vi "Read U8 Array.vi"(8 "error in":errorcluster, 9 "size":i32, 10 "register name":string, 11 "session in":u32) -> (0 "error out":errorcluster, 2 "Value out":u8[](array[numeric]), 3 "session out":u32)   [LabVIEW 2020, in "FPGA Register IO.lvlib"]
uses:
  FPGA Register IO.lvlib
  SubVIs/Check Register Data Store.vi
  Error Handling/Error 6001.vi
  Error Handling/Error 6000.vi
  Error Handling/Error 6002.vi
  NiFpga.dll
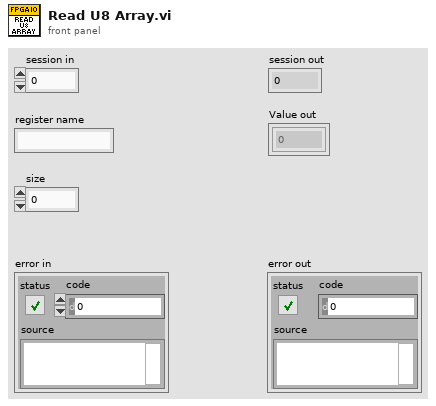
[diagram p1: front panel]
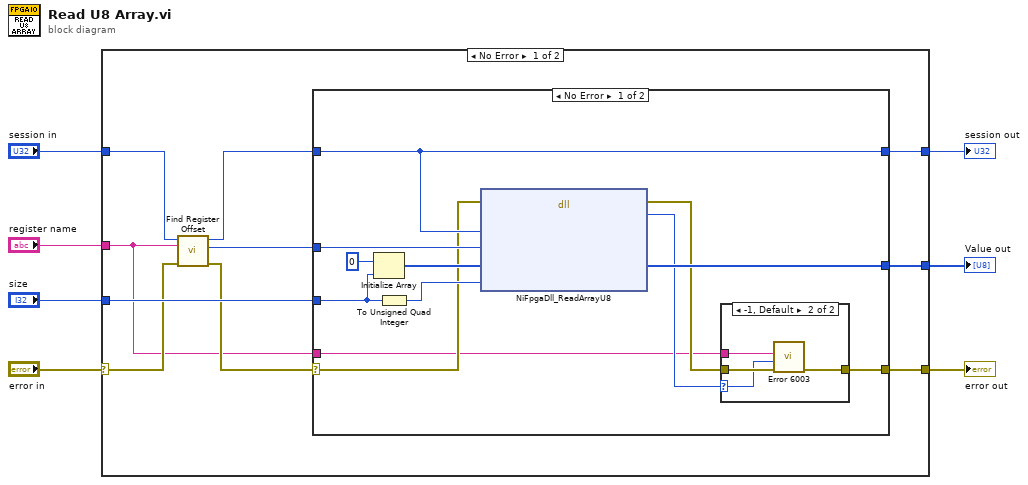
[diagram p0: block diagram]
diagram:
  n1 = case shown="No Error" "error in" {
    selector: "error in" -> [w9 w37]
    tunnel: [w17 w37] -> w7
    tunnel: [w16 w38] -> w6
    tunnel: "size" -> [w15 _]
    tunnel: [w14 _] -> w4
    tunnel: "session in" -> [w13 w38]
    tunnel: "register name" -> [w8 _]
    frame No Error {
      n2 = call "Find Register Offset.vi"("error in (no error)"=w9, "register name"=w8, "session in"=w13) -> ("error out"=w10:errorcluster, "resource offset"=w11:u32, "session out"=w12:u32)  [unwired: 6 in]
      n3 = case shown="No Error" w10 {
        selector: w10 -> [w22 w36]
        tunnel: w12 -> [w26 w35]
        tunnel: [w21 w36] -> w17
        tunnel: w11 -> [w25 _]
        tunnel: [w26 w35] -> w16
        tunnel: w15 -> [w24 _]
        tunnel: [w23 _] -> w14
        tunnel: w8 -> [w18 _]
        frame No Error {
          n4 = Initialize Array(u8 0, w24) -> (w28:u8[])
          n5 = To Unsigned Quad Integer(1:w24) -> (0:w29:u64)
          n6 = dll-call lib="NiFpga.*" fn="NiFpgaDll_ReadArrayU8"(error in=w22, "session"=w26, "offset"=w25, "data"=w28, "count"=w29) -> (error out=w20:errorcluster, "status"=w19:i32, "data"=w23:u8[])  [unwired: 5 in, 1 out]
          n7 = case shown="-1, Default" w19 {
            selector: w19 -> [_ w31]
            tunnel: w20 -> [w30 w34]
            tunnel: [w30 w33] -> w21
            tunnel: w18 -> [_ w32]
            frame 0 {
            }
            frame -1, Default {
              n8 = call "Error 6003.vi"("error in (no error)"=w34, "rio status code"=w31, "register name"=w32) -> ("error out"=w33:errorcluster)  [unwired: 8 in]
            }
          }
        }
        frame Error {
        }
      }
    }
    frame Error {
    }
  }
  "error out" <- w7
  "session out" <- w6
  "Value out" <- w4
